vi "Largest Channel Array.vi"(8 "error in (no error)":errorcluster, 10 "largest channel array in (0)":u64, 11 "Transfer in":refnum<class "Transfer.lvclass">) -> (0 "error out":errorcluster, 2 "largest channel array out":u64, 3 "Transfer out":refnum<class "Transfer.lvclass">)   [LabVIEW 2017, in "DSF Core.lvlib" / "Transfer.lvclass"]
uses:
  Transfer.lvclass
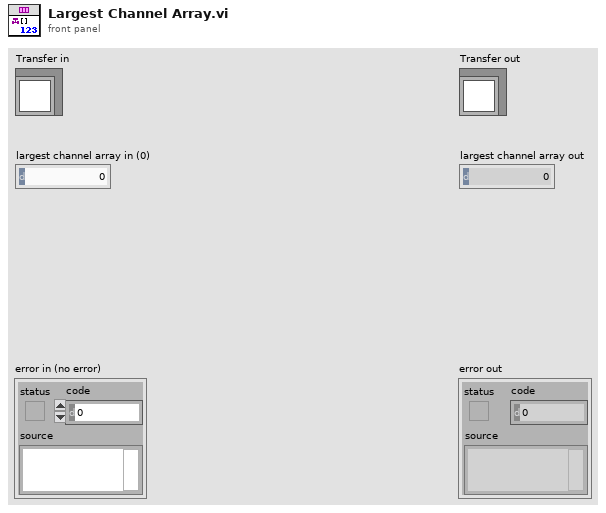
[diagram p1: front panel]
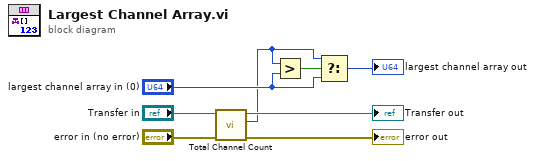
[diagram p0: block diagram]
diagram:
  n1 = call "Total Channel Count.vi"("error in (no error)"="error in (no error)", "Transfer in"="Transfer in") -> ("error out"=→"error out":errorcluster, "total channel count"=w1:u64, "Transfer out"=→"Transfer out":refnum<class "Transfer.lvclass">)  [unwired: 7 in]
  n2 = Greater?(x=w1, y="largest channel array in (0)") -> (0:w8:bool)
  n3 = Select(t=w1, s=w8, f="largest channel array in (0)") -> (s? t:f=→"largest channel array out":u64)
